vi "CRYUpdate State Variable.vi"(0 "Step VI No In":i32, 9 "Step Index":i32, 11 "Steps":T1[](array[typedef]) {"Repeat State Array"."Start" format="%#_5g"; "Y dB ref" format="%.1f"; "Y data" items=["dB", "Lin"]; "Start" format="%#_5g"}) -> (4 "Step VI No Out":i32)   [LabVIEW 2013]
uses:
  Typedef Control/CRYStep.ctl
  CRYProject Run Control Global.vi
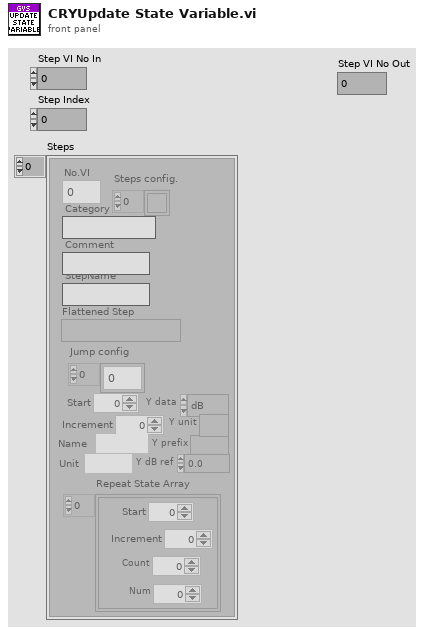
[diagram p1: front panel]
types:
  T1 = typedef "CRYStep.ctl" = cluster{"No.VI":i32, "Category":string, "StepName":string, "Seq setup flattened":string, "Comment":string, "Steps config.":bool[], "Jump config":i32[], "Start":dbl, "Increment":dbl, "Name":string, "Unit":string, "Y data":u16, "Y prefix":string, "Y dB ref":dbl, "Y unit":string, "Repeat State Array":cluster{"Start":dbl, "Increment":dbl, "Count":i32, "Num":i32}[]}
  T2 = cluster{"Start":dbl, "Increment":dbl, "Count":i32, "Num":i32}[]
  T3 = cluster{"Start":dbl, "Increment":dbl, "Count":i32, "Num":i32}
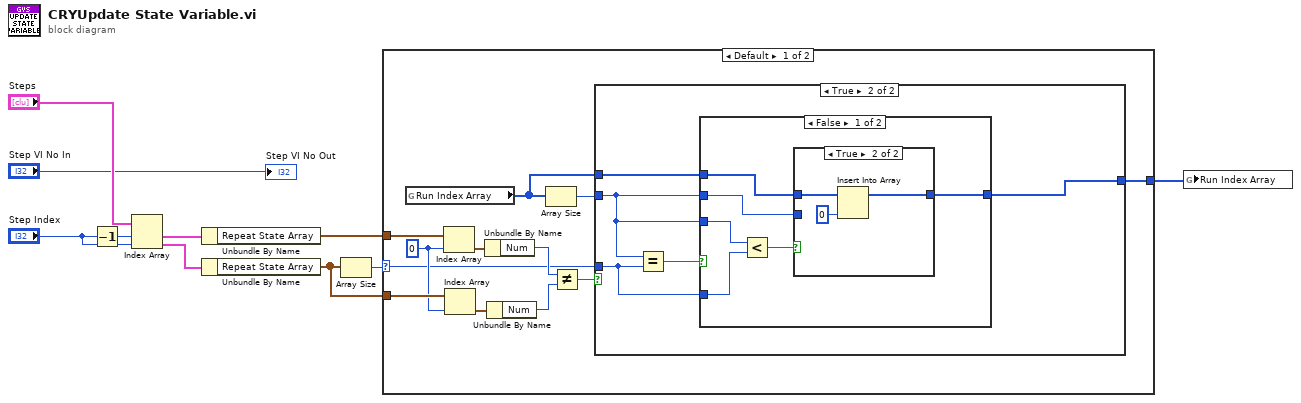
[diagram p0: block diagram]
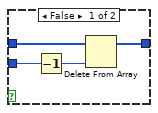
[diagram p3: hidden frame]
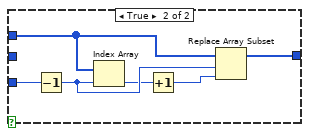
[diagram p4: hidden frame]
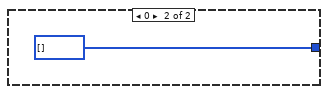
[diagram p5: hidden frame]
diagram:
  n1 = Decrement(x="Step Index") -> (x-1=w7:i32)
  n2 = Index Array(array="Steps", index #1=w7, index #2="Step Index") -> (element #1=w5:T1, element #2=w6:T1)
  n3 = Unbundle By Name(w5) -> ("Repeat State Array"=w4:T2)
  n4 = Unbundle By Name(w6) -> ("Repeat State Array"=w3:T2)
  n5 = Array Size(array=w3) -> (size(s)=w10:i32)
  n6 = case shown="Default" w10 {
    selector: w10 -> [w14 _]
    tunnel: [w12 u32[] [] ("Run Index Array")] -> w2
    tunnel: w4 -> [w22 _]
    tunnel: w3 -> [w21 _]
    frame Default {
      w20 = 0 ("index")
      n7 = global read "CRYProject Run Control Global.vi" "Run Index Array"() -> (w11:u32[])
      n8 = Index Array(array=w22, index=w20) -> (element=w19:T3)
      n9 = Index Array(array=w21, index=w20) -> (element=w18:T3)
      n10 = Unbundle By Name(w19) -> ("Num"=w17:i32)
      n11 = Unbundle By Name(w18) -> ("Num"=w16:i32)
      n12 = Array Size(array=w11) -> (size(s)=w13:i32)
      n13 = Not Equal?(x=w17, y=w16) -> (x != y?=w15:bool)
      n14 = case shown="True" w15 {
        tunnel: w14 -> [_ w25]
        tunnel: w13 -> [_ w24]
        tunnel: w11 -> [w23 w28]
        tunnel: [w23 w26] -> w12
        frame False {
        }
        frame True {
          n15 = Equal?(x=w24, y=w25) -> (x = y?=w27:bool)
          n16 = case shown="False" w27 {
            tunnel: w24 -> [w32 w47]
            tunnel: w28 -> [w34 w46]
            tunnel: [w33 w42] -> w26
            tunnel: w25 -> [w31 _]
            tunnel: w24 -> [w29 _]
            frame False {
              n17 = Less?(x=w32, y=w31) -> (x < y?=w30:bool)
              n18 = case shown="True" w30 {
                tunnel: w34 -> [w38 w41]
                tunnel: [w37 w40] -> w33
                tunnel: w29 -> [w36 _]
                frame False {
                  n19 = Decrement(x=w36) -> (x-1=w35:i32)
                  n20 = Delete From Array(array=w38, index=w35) -> (array with subset deleted=w37:u32[])  [unwired: 1 in, 1 out]
                }
                frame True {
                  n21 = Insert Into Array(array=w41, new element=u32 0 ("new element/subarray")) -> (w40:u32[])  [unwired: 1 in]
                }
              }
            }
            frame True {
              n22 = Decrement(x=w47) -> (x-1=w45:i32)
              n23 = Index Array(array=w46, index=w45) -> (element=w44:u32)
              n24 = Increment(x=w44) -> (x+1=w43:u32)
              n25 = Replace Array Subset(array=w46, new element=w43, index=w45) -> (w42:u32[])
            }
          }
        }
      }
    }
    frame 0 {
    }
  }
  n26 = global write "CRYProject Run Control Global.vi" "Run Index Array"(w2) -> ()
  "Step VI No Out" <- "Step VI No In"
